vi "Initialize Core.vi"(8 "error in":errorcluster, 10 "Shared Resources":refnum<class "Shared Resources.lvclass">, 11 "Rx Execution Unit in":refnum<class "Rx Execution Unit.lvclass">) -> (0 "error out":errorcluster, 3 "Rx Execution Unit out":refnum<class "Rx Execution Unit.lvclass">)   [LabVIEW 2020, in "AIM ARINC 429 Engine.lvlib" / "Implementation.lvlib" / "Rx Execution Unit.lvclass"]
uses:
  Rx Execution Unit.lvclass
  Hardware API/AIM ARINC 429 Hardware API.lvlib
  Shared Resources/Shared Resources.lvclass
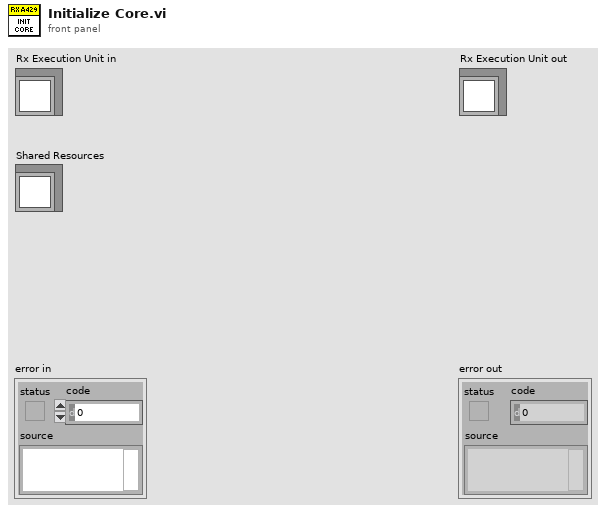
[diagram p1: front panel]
types:
  T1 = typedef "RT Hardware Channel Settings.ctl" = cluster{"channel #":u16, "channel handle":u64, "labels settings for RT":T2[], "speed":T10}
  T2 = typedef "RT Label Settings.ctl" = cluster{"Name":string, "xmlName":string, "label":T3, "transfer period":u32, "SDI_Enabled":bool, "SDI":u8, "parameter driver data":T4, "transfer type":T8, "has timestamp?":bool, "Label Disable/Trigger Channel Reference":T7, "Message Handle":u64, "Initialized?":bool, "Word Initial Raw Value":u32, "Label Timestamp Channel Data Reference":T9, "disabled":bool, "modified":bool}
  T3 = typedef "Label.ctl" = u8
  T4 = typedef "RT Parameters.ctl" = cluster{"parameter definitions":T5[], "Tx parameter refs":T7[]}
  T5 = typedef "Parameter Definition.ctl" = cluster{"start index":i32, "size":i32, "encoding":T6, "signed":bool, "scale multiplier":dbl, "scale offset":dbl, "default value":dbl}
  T6 = typedef "Encoding and Decoding.lvlib/Encoding.ctl" = enum16{"BNR", "BCD", "Discrete"}
  T7 = typedef "Custom Device API.lvlib/Custom Device Item Ref.ctl" = u64
  T8 = typedef "Transfer Type.ctl" = enum16{"Scheduled", "Acyclic", "Block", "Strobe"}
  T9 = typedef "Custom Device API.lvlib/Data Reference.ctl" = i32
  T10 = typedef "Transfer Speed.ctl" = enum16{"LO (12.5 kb/s)", "HI (100 kb/s)"}
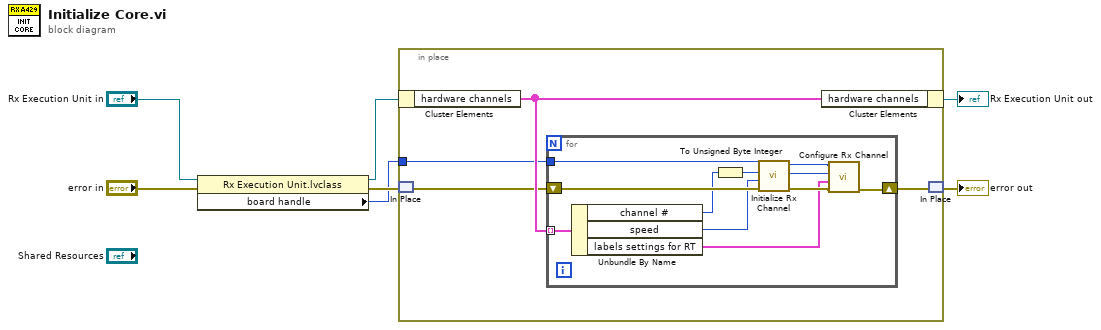
[diagram p0: block diagram]
diagram:
  n1 = property class="Rx Execution Unit.lvclass"(reference="Rx Execution Unit in", error in="error in") -> (reference out=w3:refnum<class "Rx Execution Unit.lvclass">, error out=w4:errorcluster, "board handle"=w1:u8)
  n2 = in-place {
    in-place-border: w1 -> [w8]
    n3 = in-place-cluster #1(w3) -> ("hardware channels"=w11:T1[])
    n4 = in-place-match #2(w4) -> (w10:errorcluster)
    n5 = for {
      tunnel: w11 -> [w22] mode=indexing
      shift-right: [w14] -> w9
      shift-left: w10 -> [w21]
      tunnel: w8 -> [w18]
      n6 = Unbundle By Name(w22) -> ("channel #"=w20:u16, "speed"=w13:T10, "labels settings for RT"=w12:T2[])
      n7 = To Unsigned Byte Integer(number=w20) -> (unsigned 8bit integer=w19:u8)
      n8 = call "Initialize Rx Channel.vi"("error in"=w21, "channel speed"=w13, "channel number"=w19, "board handle"=w18) -> ("error out"=w15:errorcluster, "channel number out"=w16:u8, "board handle out"=w17:u8)  [unwired: 5 in]
      n9 = call "Configure Rx Channel.vi"("error in"=w15, "labels settings for RT"=w12, "channel number in"=w16, "board handle in"=w17) -> ("error out"=w14:errorcluster)  [unwired: 5 in, 2 out]
    }
    n10 = in-place-cluster #1("hardware channels"=w11) -> (→"Rx Execution Unit out":refnum<class "Rx Execution Unit.lvclass">)
    n11 = in-place-match #2(w9) -> (→"error out":errorcluster)
  }
